vi "Add.vi"(8 "error in (no error)":errorcluster, 9 "Value":variant, 10 "Key":string, 11 "Dictionary in":refnum<class "Dictionary.lvclass">) -> (0 "error out":errorcluster, 1 "Success?":bool, 3 "Dictionary out":refnum<class "Dictionary.lvclass">)   [LabVIEW 2018, in "Application.lvlib" / "Dictionary.lvclass"]
uses:
  Dictionary.lvclass
  Dictionary.lvclass/Dictionary.ctl
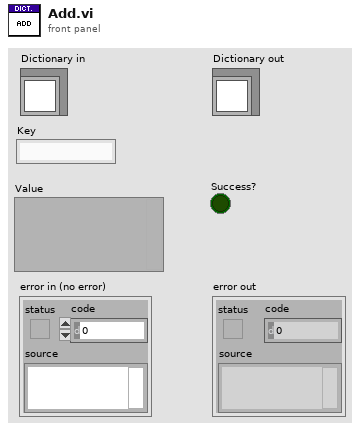
[diagram p1: front panel]
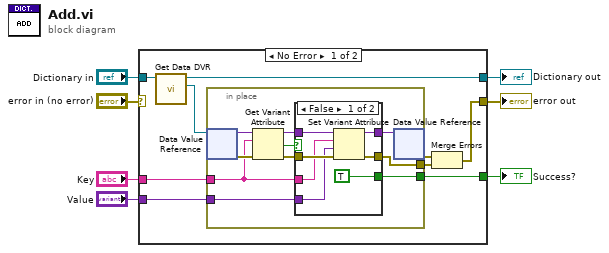
[diagram p0: block diagram]
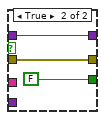
[diagram p2: hidden frame]
diagram:
  n1 = case shown="No Error" "error in (no error)" {
    selector: "error in (no error)" -> [_ w38]
    tunnel: [w8 w38] -> w6
    tunnel: [w12 w37] -> w4
    tunnel: "Dictionary in" -> [w16 w37]
    tunnel: "Key" -> [w14 _]
    tunnel: "Value" -> [w13 _]
    tunnel: [w11 _] -> w1
    frame No Error {
      n2 = call "Get Data DVR.vi"("Dictionary in"=w16) -> ("Data DVR"=w15:refnum<data-value>, "Dictionary out"=w12:refnum<class "Dictionary.lvclass">)  [unwired: 8 in, 1 out]
      n3 = in-place {
        in-place-border: w13 -> [w18]
        in-place-border: w14 -> [w19]
        in-place-border: [w20] -> w11
        in-place-border: [w17] -> w9
        n4 = in-place-dvr #1(w15) -> (w22:variant, w23:errorcluster)
        n5 = Get Variant Attribute(Variant=w22, name=w19, error in=w23) -> (duplicate Variant=w26:variant, found=w25:bool, error out=w24:errorcluster)  [unwired: 1 in, 1 out]
        n6 = case shown="False" w25 {
          tunnel: [w33 w35] -> w17
          tunnel: [w32 w36] -> w21
          tunnel: [TRUE FALSE] -> w20
          tunnel: w26 -> [w31 w36]
          tunnel: w24 -> [w30 w35]
          tunnel: w19 -> [w29 _]
          tunnel: w18 -> [w28 _]
          frame False {
            n7 = Set Variant Attribute(Variant=w31, name=w29, value=w28, error in=w30) -> (Variant out=w32:variant, error out=w33:errorcluster)  [unwired: 1 out]
          }
          frame True {
          }
        }
        n8 = in-place-dvr #1(w21) -> (w10:errorcluster)  [unwired: 1 out]
      }
      n9 = Merge Errors(w10, w9) -> (w8:errorcluster)
    }
    frame Error {
    }
  }
  "error out" <- w6
  "Dictionary out" <- w4
  "Success?" <- w1
